vi "FRCts20_Backend_Team_DELETE.vi"(6 "Message Attributes":T4, 8 "error in (no error)":errorcluster, 10 "Data":string, 11 "Engine_Refnums":T1) -> (0 "error out":errorcluster)   [LabVIEW 2014, in "FRCts20_Backend_Engine.lvlib"]
doc: "Deletes a team, but does not delete requests which are children of the team. Called by the Team API, expects a team index."
uses:
  FRCts20_Backend_Engine.lvlib
  Dependencies/Keyed Array/KeyedArray.ctl
  FRCts20_Backend_EngineRefnums.ctl
  INI_Accessor/FRCts20_Backend_INI Controller.lvclass
  Dependencies/AMC/_SubVIs/TypeDefs/Message Queue.ctl
  Dependencies/AMC/_SubVIs/TypeDefs/Message.ctl
  <vilib>/addons/database/Connection.llb/Conn ObjectReference.ctl
  FRCts20_Backend_FGVOperation.ctl
  FRCts20_Backend_API/FRCts20_Backend_API_Status.ctl
  FRCts20_Backend_API/FRCts20_Backend_API.lvlib
  FRCts20_Backend_API/FRCts20_Backend_API_Team.ctl
  FRCts20_Backend_API/FRCts20_Backend_API_SW.ctl
  Dependencies/Keyed Array/Tools_KeyedArray.lvlib
  Dependencies/AMC/AMC.lvlib
  <vilib>/addons/database/NI_Database_API.lvlib
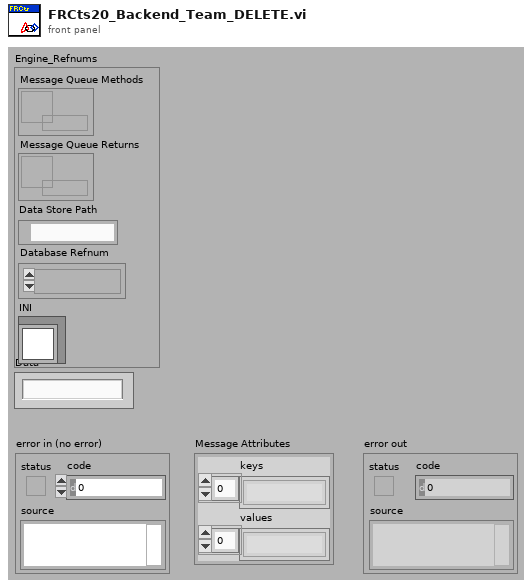
[diagram p1: front panel]
types:
  T1 = typedef "FRCts20_Backend_Engine.lvlib/FRCts20_Backend_EngineRefnums.ctl" = cluster{"Message Queue Methods":T2, "Message Queue Returns":T2, "Data Store Path":path, "Database Refnum":T3, "INI":refnum<class "FRCts20_Backend_INI Controller.lvclass">}
  T2 = typedef "AMC.lvlib/Message Queue.ctl" = refnum<queue>
  T3 = typedef "NI_Database_API.lvlib/Conn ObjectReference.ctl" = refnum<k1>
  T4 = typedef "Tools_KeyedArray.lvlib/KeyedArray.ctl" = cluster{"keys":string[], "values":string[]}
  T5 = typedef "FRCts20_Backend_Engine.lvlib/FRCts20_Backend_API.lvlib/FRCts20_Backend_API_Team.ctl" = cluster{"Team Index":u32, "Team Number":u32, "Team Name":string, "Short Team Name":string, "Nick Name":string, "Robot Name":string, "City":string, "State":string, "Country":string, "Rookie Year":u32, "SWType":T6, "CAN":bool, "Vision":bool, "Kinect":bool, "Tags":string, "Avatar":string, "Request Array":cluster{"Request Index":u32, "Description":string, "Status":T7, "Open Date":timestamp, "Last Update":timestamp, "Close Date":timestamp}[], "Events Attending":cluster{"EventIndex":i32, "EventName":string, "IsLive":bool}[], "APIReturn":string}
  T6 = typedef "FRCts20_Backend_Engine.lvlib/FRCts20_Backend_API.lvlib/FRCts20_Backend_API_SW.ctl" = string
  T7 = typedef "FRCts20_Backend_Engine.lvlib/FRCts20_Backend_API.lvlib/FRCts20_Backend_API_Status.ctl" = i32
  T8 = typedef "FRCts20_Backend_Engine.lvlib/FRCts20_Backend_FGVOperation.ctl" = enum16{"Initialize", "EnqueueMessage", "EnqueueDataReturn", "FlushMessage", "FlushDataReturn"}
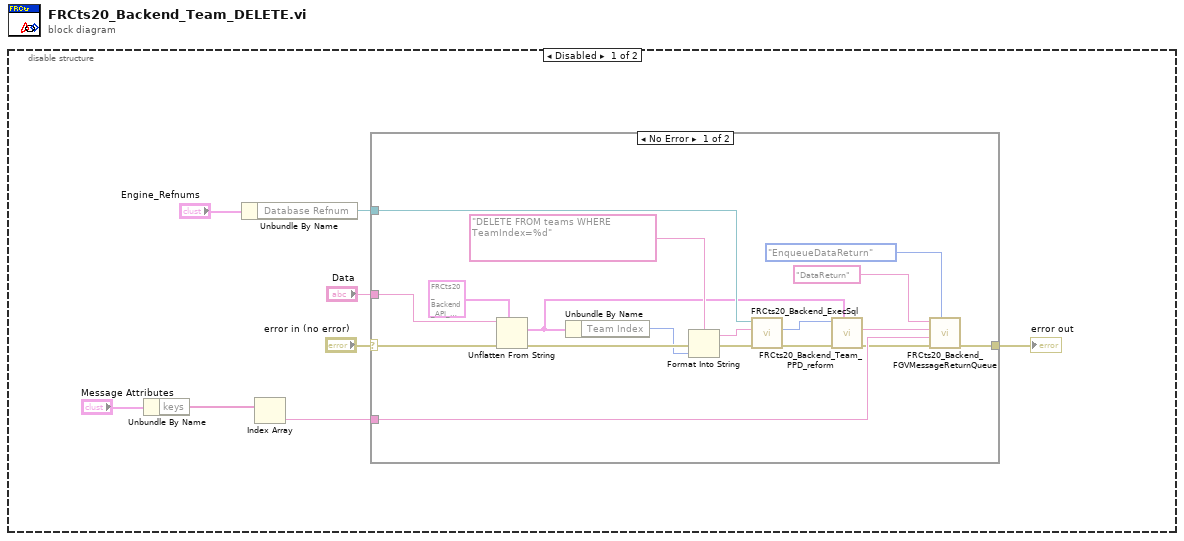
[diagram p0: block diagram]
diagram:
  n1 = disable-structure shown="Disabled" {
    frame Disabled {
      n2 = Unbundle By Name("Message Attributes") -> ("keys"=w2:string[])
      n3 = Unbundle By Name("Engine_Refnums") -> ("Database Refnum"=w5:T3)
      n4 = Index Array(array=w2) -> (element=w1:string)  [unwired: 1 in]
      n5 = case shown="No Error" "error in (no error)" {
        selector: "error in (no error)" -> [w23 w27]
        tunnel: [w26 w27] -> w7
        tunnel: w5 -> [w15 _]
        tunnel: "Data" -> [w24 _]
        tunnel: w1 -> [w25 _]
        frame No Error {
          n6 = Unflatten From String(type=T5 {"Team Index"=0, "Team Number"=0, "Team Name"="", "Short Team Name"="", "Nick Name"="", "Robot Name"="", "City"="", "State"="", "Country"="", "Rookie Year"=0, "SWType"="", "CAN"=FALSE, "Vision"=FALSE, "Kinect"=FALSE, "Tags"="", "Avatar"="", "Request Array"=[], "Events Attending"=[], "APIReturn"=""} ("Team"), binary string=w24, error in (no error)=w23) -> (value=w11:T5, error out=w22:errorcluster)  [unwired: 2 in, 1 out]
          n7 = Unbundle By Name(w11) -> ("Team Index"=w20:u32)
          n8 = Format Into String(format string="DELETE FROM teams WHERE TeamIndex=%d", error in=w22, w20) -> (resulting string=w14:string, error out=w16:errorcluster)  [unwired: 1 in]
          n9 = call "FRCts20_Backend_ExecSql.vi"("error in (no error)"=w16, "format string"=w14, "Refnum in"=w15) -> ("error out"=w13:errorcluster, "rows affected"=w12:i32)  [unwired: 6 in, 1 out]
          n10 = call "FRCts20_Backend_Team_PPD_reform.vi"("TeamRoot"=w11, "error in (no error)"=w13, "rows affected"=w12) -> ("error out"=w9:errorcluster, "data string"=w10:string)  [unwired: 7 in]
          n11 = call "FRCts20_Backend_FGVMessageReturnQueue.vi"("Operation"=FRCts20_Backend_FGVOperation."EnqueueDataReturn", "error in (no error)"=w9, "Key"=w25, "Message Value"=w10, "Message Name"="DataReturn") -> ("error out"=w26:errorcluster)  [unwired: 5 in, 1 out]
        }
        frame Error {
        }
      }
      "error out" <- w7
    }
    frame Enabled {
    }
  }
